vi "Grava_summaryEQ.vi"(1 "summary EQ":string, 3 "quants pixels bons per Chip":u8[](array[numeric]), 4 "ChipID list":u32[](array[numeric]) format="%x", 5 "file name":string, 6 "subfolder path: text reports":path) -> ()   [LabVIEW 2015, in "VIPM2.lvlib"]
doc: "Grava arxiu de text amb resum de pixels bons per ChipID.\nAl final s'afageix el EQ summary."
uses:
  VIPM2.lvlib
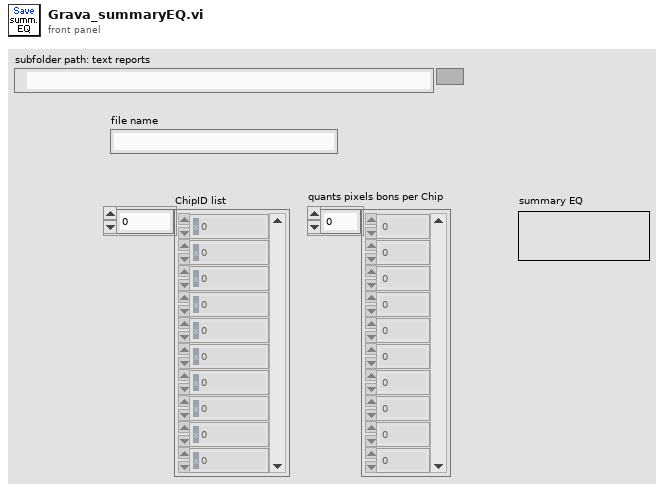
[diagram p1: front panel]
types:
  T1 = enum16{"open", "replace", "create", "open or create", "replace or create", "replace or create with confirmation"}
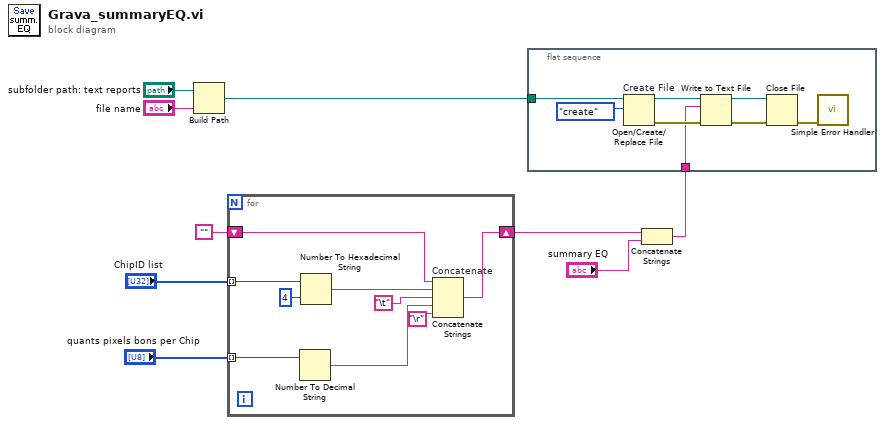
[diagram p0: block diagram]
diagram:
  n1 = Build Path(base path="subfolder path: text reports", name or relative path="file name") -> (appended path=w9:path)
  n2 = for {
    tunnel: "ChipID list" -> [w18] mode=indexing
    tunnel: "quants pixels bons per Chip" -> [w16] mode=indexing
    shift-right: [w10] -> w3
    shift-left: "" -> [w11]
    n3 = Number To Decimal String(number=w16) -> (decimal integer string=w13:string)  [unwired: 1 in]
    n4 = Number To Hexadecimal String(1:i16 4 ("width (-)"), 2:w18) -> (0:w15:string)
    n5 = Concatenate Strings "Concatenate"(w11, w15, "\t", w13, "\r") -> (w10:string)
  }
  n6 = flat-sequence {
    tunnel: w9 -> [w26]
    tunnel: w2 -> [w19]
    frame #0 {
      n7 = Open/Create/Replace File "Create File"(file path (use dialog)=w26, operation (0:open)=T1."create") -> (refnum out=w24:refnum<file>, error out=w23:errorcluster)  [unwired: 4 in, 1 out]
      n8 = Write to Text File(file (use dialog)=w24, text=w19, error in=w23) -> (refnum out=w22:refnum<file>, error out=w21:errorcluster)  [unwired: 1 in, 1 out]
      n9 = Close File(refnum=w22, error in=w21) -> (error out=w20:errorcluster)  [unwired: 1 out]
      n10 = call <vilib>:"Simple Error Handler.vi"("error in (no error)"=w20) -> ()  [unwired: 4 in, 5 out]
    }
  }
  n11 = Concatenate Strings "Concatenate Strings"(w3, "summary EQ") -> (w2:string)
